vi "Chapet3_Triangular_waveform.vi"() -> ()   [LabVIEW 2013]
panel:
  in  "stop":bool
  out "data":dynamicdata(graph)
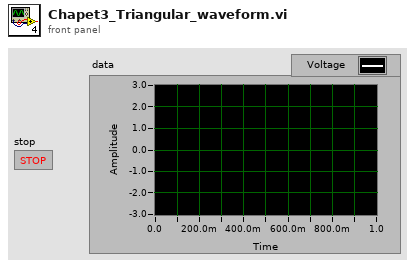
[diagram p1: front panel]
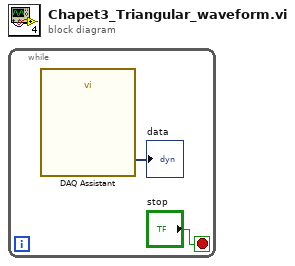
[diagram p0: block diagram]
diagram:
  n1 = while {
    stop <- "stop" stop-if-true
    n2 = call "DAQ Assistant"() -> ("data"=→"data":dynamicdata)  [unwired: 17 in, 2 out]
  }
